vi "brush.vi"(7 "colorGroup (All)":T2=5 items=["Active"=0, "Disabled"=1, "Inactive"=2, "All"=5], 8 "Error In":errorcluster, 10 "colorRole (NoRole)":T1=17 items=["WindowText", "Button", "Light", "Midlight", "Dark", "Mid", "Text", "BrightText", "ButtonText", "Base", "Window", "Shadow", "Highlight", "HighlightedText", "Link", "LinkVisited", "AlternateBase", "NoRole", "ToolTipBase", "ToolTipText", "PlaceholderText"], 11 "QPalette In":refnum<class "QPalette.lvclass">) -> (0 "Error Out":errorcluster, 2 "Value":refnum<class "QBrush.lvclass">, 3 "QPalette Out":refnum<class "QPalette.lvclass">)   [LabVIEW 2014, in "QPalette.lvclass"]
doc: "LabVIEW-specific documentation is not yet available. See <b>https://doc.qt.io/qt-5/qpalette.html#brush</b>"
uses:
  QPalette.lvclass
  QBrush/QBrush.lvclass
  ColorGroup.ctl
  ColorRole.ctl
  LQ Core/LQSerialData/LQSerialData.lvclass/LQSerialData.ctl
  LQ Core/LQ Core.lvlib
  LQ Core/LQSerialData/LQSerialData.lvclass
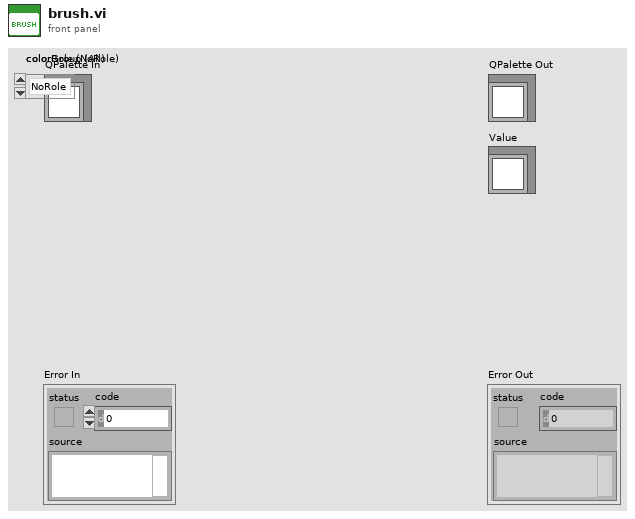
[diagram p1: front panel]
types:
  T1 = typedef "QPalette.lvclass/ColorRole.ctl" = i32
  T2 = typedef "QPalette.lvclass/ColorGroup.ctl" = i32
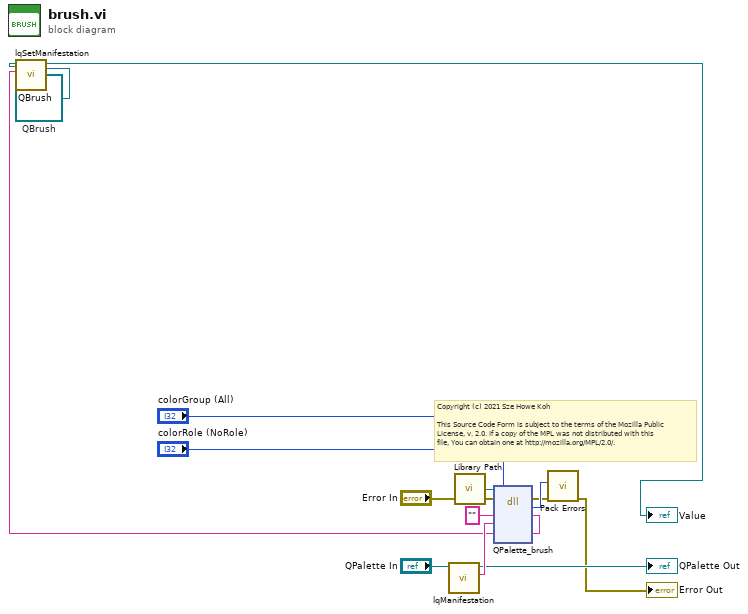
[diagram p0: block diagram]
diagram:
  w3 = refnum<class "QBrush.lvclass"> refnum  # QBrush
  # "Copyright (c) 2021 Sze Howe Koh\n\nThis Source Code Form is subject to the terms of the Mozilla Public\nLicense, v. 2.0. If a copy of the MPL was not distributed with this\nfile, You can obtain one at http://mozilla.org/MPL/2.0/."
  n1 = call "lqManifestation.vi"("LQSerialData in"="QPalette In") -> ("Manifestation"=w12:string, "LQSerialData out"=→"QPalette Out":refnum<class "QPalette.lvclass">)  [unwired: 9 in]
  n2 = call "Library Path.vi"() -> ("Library Path"=w9:path)
  n3 = dll-call lib="?" fn="QPalette_brush"(path in=w9, error in="Error In", "_retVal"="" ("retVal"), "_instance"=w12, "colorGroup"="colorGroup (All)", "colorRole"="colorRole (NoRole)") -> (error out=w7:errorcluster, w8:i32, "_retVal"=w4:string)  [unwired: 4 in, 1 out]
  n4 = call "lqSetManifestation.vi"("Manifestation"=w4, "LQSerialData in"=w3) -> ("LQSerialData out"=→"Value":refnum<class "QBrush.lvclass">)  [unwired: 8 in, 1 out]
  n5 = call "Pack Errors.vi"("Error In"=w7, "Error Code"=w8) -> ("Error Out"=→"Error Out":errorcluster)  [unwired: 9 in]
